vi "UpdateCCDconf.vi"(8 "error in (no error)":errorcluster, 10 "status":string, 11 "Interface in":refnum<class "Interface.lvclass">) -> (0 "error out":errorcluster, 1 "CCD conf rx":T1, 2 "Cluster comparison":T2, 3 "Interface out":refnum<class "Interface.lvclass">)   [LabVIEW 2018, in "Interface.lvclass"]
uses:
  Interface.lvclass
panel:
  in  "Cluster CCD conf":cluster{"CCD configuration":string}
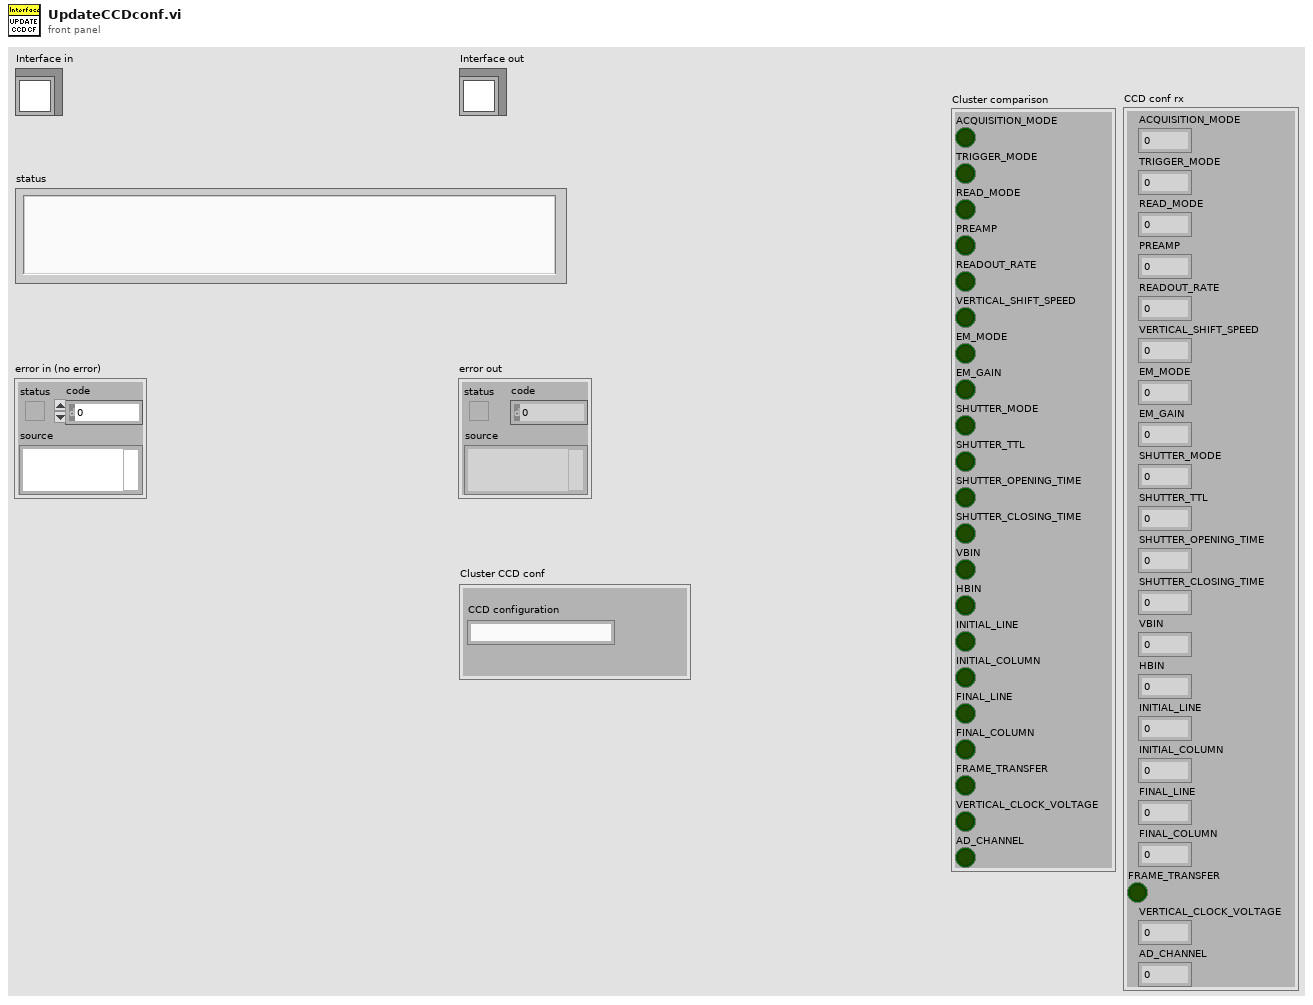
[diagram p1: front panel]
types:
  T1 = cluster{"ACQUISITION_MODE":u8, "TRIGGER_MODE":u8, "READ_MODE":u8, "PREAMP":u8, "READOUT_RATE":u8, "VERTICAL_SHIFT_SPEED":u8, "EM_MODE":u8, "EM_GAIN":u16, "SHUTTER_MODE":u8, "SHUTTER_TTL":u8, "SHUTTER_OPENING_TIME":u16, "SHUTTER_CLOSING_TIME":u16, "VBIN":u16, "HBIN":u16, "INITIAL_LINE":u16, "INITIAL_COLUMN":u16, "FINAL_LINE":u16, "FINAL_COLUMN":u16, "FRAME_TRANSFER":bool, "VERTICAL_CLOCK_VOLTAGE":u8, "AD_CHANNEL":u32}
  T2 = cluster{"ACQUISITION_MODE":bool, "TRIGGER_MODE":bool, "READ_MODE":bool, "PREAMP":bool, "READOUT_RATE":bool, "VERTICAL_SHIFT_SPEED":bool, "EM_MODE":bool, "EM_GAIN":bool, "SHUTTER_MODE":bool, "SHUTTER_TTL":bool, "SHUTTER_OPENING_TIME":bool, "SHUTTER_CLOSING_TIME":bool, "VBIN":bool, "HBIN":bool, "INITIAL_LINE":bool, "INITIAL_COLUMN":bool, "FINAL_LINE":bool, "FINAL_COLUMN":bool, "FRAME_TRANSFER":bool, "VERTICAL_CLOCK_VOLTAGE":bool, "AD_CHANNEL":bool}
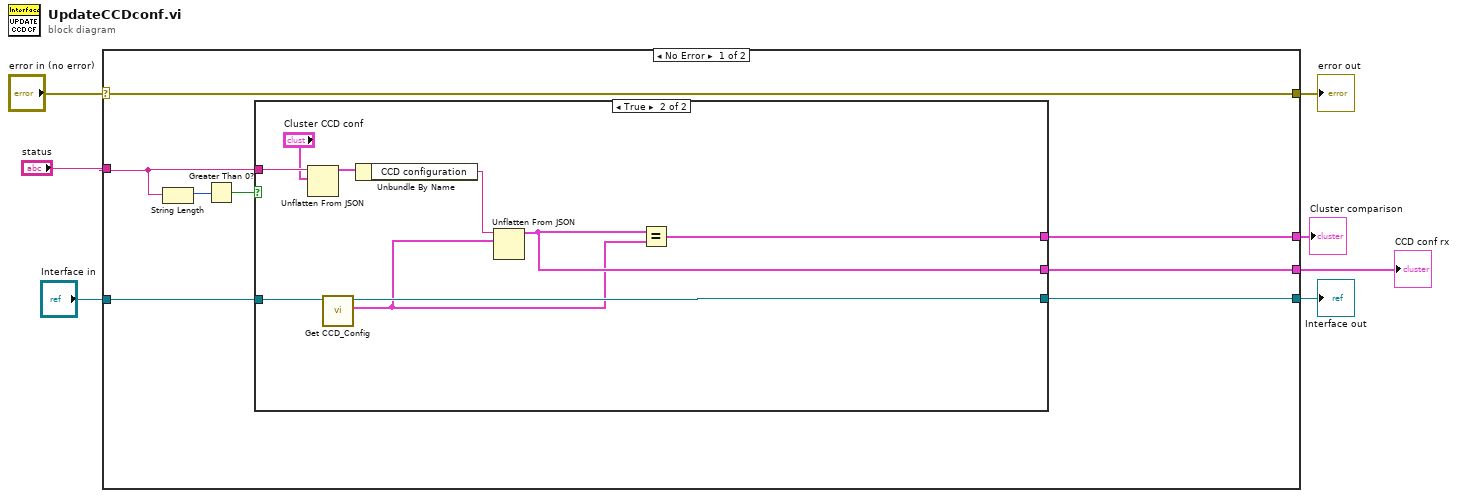
[diagram p0: block diagram]
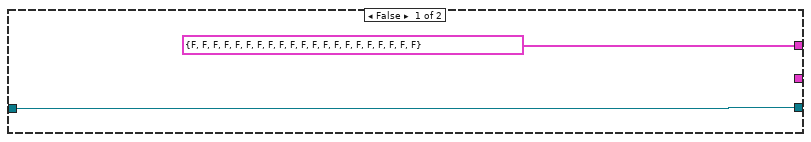
[diagram p2: hidden frame]
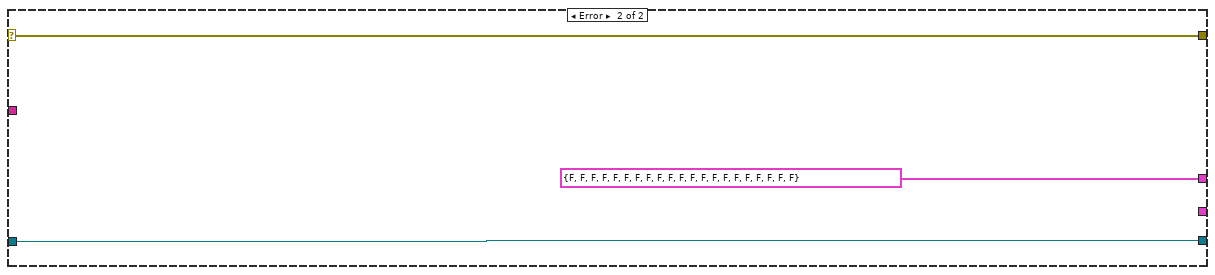
[diagram p3: hidden frame]
diagram:
  n1 = case shown="No Error" "error in (no error)" {
    selector: "error in (no error)" -> [w15 w29]
    tunnel: [w15 w29] -> w6
    tunnel: [w14 w28] -> w4
    tunnel: "Interface in" -> [w12 w28]
    tunnel: "status" -> [w10 _]
    tunnel: [w9 T2 {"ACQUISITION_MODE"=FALSE, "TRIGGER_MODE"=FALSE, "READ_MODE"=FALSE, "PREAMP"=FALSE, "READOUT_RATE"=FALSE, "VERTICAL_SHIFT_SPEED"=FALSE, "EM_MODE"=FALSE, "EM_GAIN"=FALSE, "SHUTTER_MODE"=FALSE, "SHUTTER_TTL"=FALSE, "SHUTTER_OPENING_TIME"=FALSE, "SHUTTER_CLOSING_TIME"=FALSE, "VBIN"=FALSE, "HBIN"=FALSE, "INITIAL_LINE"=FALSE, "INITIAL_COLUMN"=FALSE, "FINAL_LINE"=FALSE, "FINAL_COLUMN"=FALSE, "FRAME_TRANSFER"=FALSE, "VERTICAL_CLOCK_VOLTAGE"=FALSE, "AD_CHANNEL"=FALSE}] -> w2
    tunnel: [w8 _] -> w1
    frame No Error {
      n2 = String Length(string=w10) -> (length=w13:i32)
      n3 = Greater Than 0?(x=w13) -> (x > 0?=w11:bool)
      n4 = case shown="True" w11 {
        tunnel: [w17 w21] -> w14
        tunnel: w10 -> [_ w26]
        tunnel: w12 -> [w17 w22]
        tunnel: [T2 {"ACQUISITION_MODE"=FALSE, "TRIGGER_MODE"=FALSE, "READ_MODE"=FALSE, "PREAMP"=FALSE, "READOUT_RATE"=FALSE, "VERTICAL_SHIFT_SPEED"=FALSE, "EM_MODE"=FALSE, "EM_GAIN"=FALSE, "SHUTTER_MODE"=FALSE, "SHUTTER_TTL"=FALSE, "SHUTTER_OPENING_TIME"=FALSE, "SHUTTER_CLOSING_TIME"=FALSE, "VBIN"=FALSE, "HBIN"=FALSE, "INITIAL_LINE"=FALSE, "INITIAL_COLUMN"=FALSE, "FINAL_LINE"=FALSE, "FINAL_COLUMN"=FALSE, "FRAME_TRANSFER"=FALSE, "VERTICAL_CLOCK_VOLTAGE"=FALSE, "AD_CHANNEL"=FALSE} w20] -> w9
        tunnel: [_ w19] -> w8
        frame False {
        }
        frame True {
          n5 = Unflatten From JSON(JSON string=w26, type and defaults="Cluster CCD conf") -> (value=w24:cluster{"CCD configuration":string})  [unwired: 5 in, 1 out]
          n6 = call-dynamic "Get CCD_Config.vi"("Interface in"=w22) -> ("output cluster"=w18:T1, "Interface out"=w21:refnum<class "Interface.lvclass">)  [unwired: 8 in, 1 out]
          n7 = Unbundle By Name(w24) -> ("CCD configuration"=w23:string)
          n8 = Unflatten From JSON(JSON string=w23, type and defaults=w18) -> (value=w19:T1)  [unwired: 5 in, 1 out]
          n9 = Equal?(x=w19, y=w18) -> (x = y?=w20:T2)
        }
      }
    }
    frame Error {
    }
  }
  "error out" <- w6
  "Interface out" <- w4
  "Cluster comparison" <- w2
  "CCD conf rx" <- w1
